vi "CCD Acquire Spectrum vs Wavelength.vi"(11 "error in":errorcluster) -> (15 "error out":errorcluster)   [LabVIEW 2020, in "Examples.lvlib"]
doc: "Example for a CCD spectrum acquisition."
uses:
  Examples.lvlib
  4aef6941-9f58-45d1-a797-2b486d7897ac.vi
  Classes/CCD/CCD.lvclass
  Classes/Mono/Monochromator.lvclass
  <userlib>/_OpenG.lib/error/error.llb/openg_error.lvlib
  <vilib>/Utility/file.llb/Write Delimited Spreadsheet (DBL).vi
panel:
  out "new wavelength":dbl format="%.2f"
  out "XY Graph":cluster{"xAxis":dbl[], "imageData":dbl[]}(graph)
  # "Connector Pane"
  # "Locals"
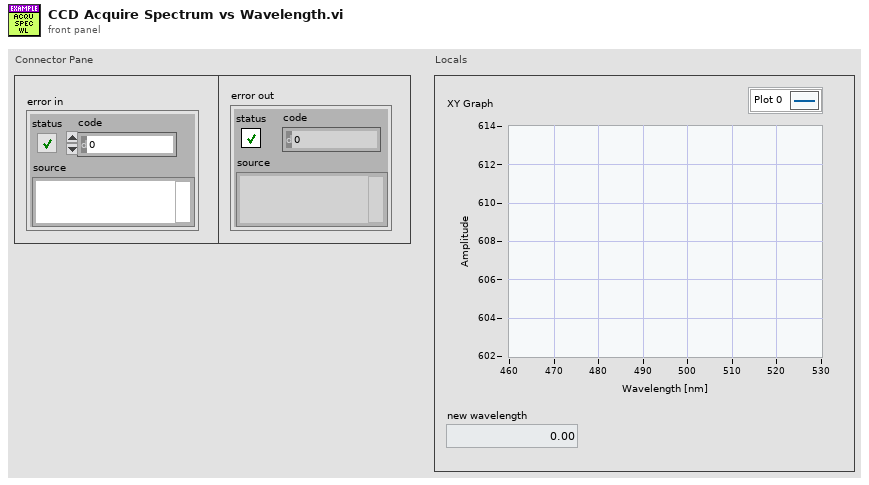
[diagram p1: front panel]
types:
  T1 = cluster{"ROI-index":i32, "xOrigin":i32, "yOrigin":i32, "xSize":i32, "ySize":i32, "xBin":i32, "yBin":i32}
  T2 = typedef "horiba.lvlib/CCD.lvclass/ccdAcquisitionData.ctl" = cluster{"acqIndex":i32, "ROIs":T3[], "timestamp":string}
  T3 = typedef "horiba.lvlib/CCD.lvclass/imageAcqData.ctl" = cluster{"roiMetaData":T4, "xAxis":dbl[], "yData":dbl[][]}
  T4 = typedef "horiba.lvlib/CCD.lvclass/roiMetaData.ctl" = cluster{"roiIndex":i32, "xBinning":i32, "xOrigin":i32, "xSize":i32, "yBinning":i32, "yOrigin":i32, "ySize":i32}
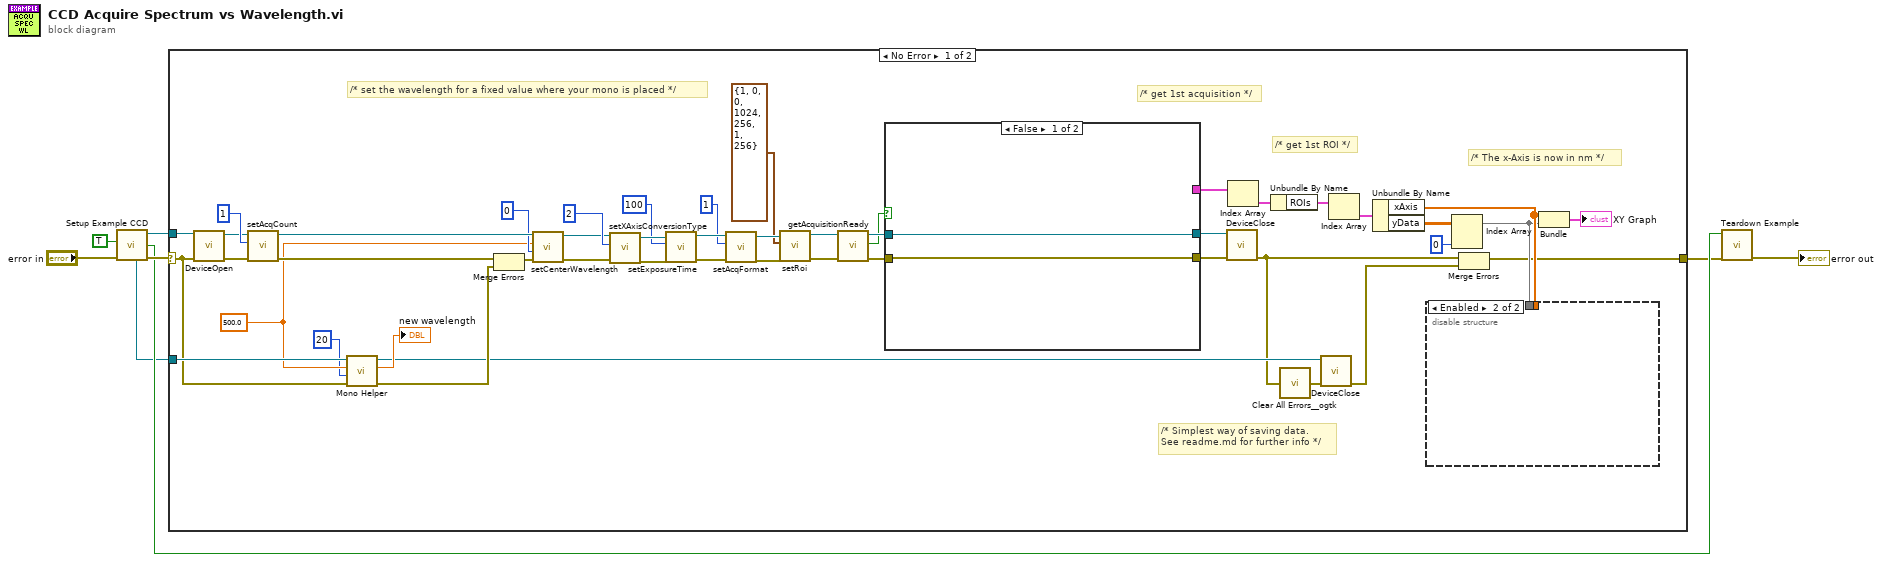
[diagram p0: block diagram]
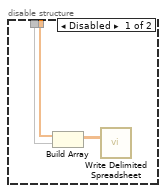
[diagram p2: hidden frame]
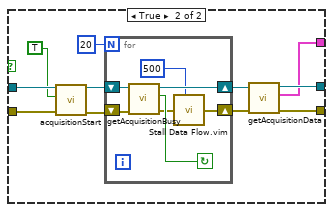
[diagram p3: hidden frame]
diagram:
  n1 = call "Setup Example CCD.vi"("error in (no error)"="error in", "show ICL for debugging"=TRUE) -> ("error out"=w6:errorcluster, "Module Was Already Running?"=w4:bool, "CCD out"=w5:refnum<class "CCD.lvclass">, "Mono out"=w1:refnum<class "Monochromator.lvclass">)  [unwired: 6 in]
  n2 = case shown="No Error" w6 {
    selector: w6 -> [w20 w79]
    tunnel: w5 -> [w32 _]
    tunnel: [w13 w79] -> w3
    tunnel: w1 -> [w21 _]
    frame No Error {
      w10 = 500.0 ("wavelength")
      # "/* set the wavelength for a fixed value where your mono is placed */"
      # "/* The x-Axis is now in nm */"
      # "/* Simplest way of saving data.\nSee readme.md for further info */"
      # "/* get 1st ROI */"
      # "/* get 1st acquisition */"
      n3 = call-dynamic "DeviceOpen.vi"("error in (no error)"=w20, "CCD in"=w32) -> ("error out"=w33:errorcluster, "CCD out"=w31:refnum<class "CCD.lvclass">)  [unwired: 6 in, 2 out]
      n4 = call "setAcqCount.vi"("error in (no error)"=w33, "count"=1, "CCD in"=w31) -> ("error out"=w18:errorcluster, "CCD out"=w26:refnum<class "CCD.lvclass">)  [unwired: 5 in, 2 out]
      n5 = call "Mono Helper.vi"("error in (no error)"=w20, "no of iterations before stop"=20, "wavelength in"=w10, "Monochromator in"=w21) -> ("error out"=w16:errorcluster, "wavelength out"=→"new wavelength":dbl, "Monochromator out"=w15:refnum<class "Monochromator.lvclass">)  [unwired: 5 in]
      n6 = Merge Errors(w18, w16) -> (w17:errorcluster)
      n7 = call "setCenterWavelength.vi"("error in (no error)"=w17, "monoIndex"=0, "wavelength"=w10, "CCD in"=w26) -> ("error out"=w27:errorcluster, "CCD out"=w25:refnum<class "CCD.lvclass">)  [unwired: 4 in, 2 out]
      n8 = call "setXAxisConversionType.vi"("error in (no error)"=w27, "type"=2, "CCD in"=w25) -> ("error out"=w53:errorcluster, "CCD out"=w52:refnum<class "CCD.lvclass">)  [unwired: 5 in, 2 out]
      n9 = call "setExposureTime.vi"("error in (no error)"=w53, "exposure time [ms] or [us]"=100, "CCD in"=w52) -> ("error out"=w50:errorcluster, "CCD out"=w49:refnum<class "CCD.lvclass">)  [unwired: 5 in, 2 out]
      n10 = call "setAcqFormat.vi"("error in (no error)"=w50, "number of ROIs"=1, "CCD in"=w49) -> ("error out"=w47:errorcluster, "CCD out"=w46:refnum<class "CCD.lvclass">)  [unwired: 5 in, 2 out]
      n11 = call "setRoi.vi"("error in (no error)"=w47, "roiConfig"=T1 {"ROI-index"=1, "xOrigin"=0, "yOrigin"=0, "xSize"=1024, "ySize"=256, "xBin"=1, "yBin"=256}, "CCD in"=w46) -> ("error out"=w45:errorcluster, "CCD out"=w28:refnum<class "CCD.lvclass">)  [unwired: 5 in, 2 out]
      n12 = call "getAcquisitionReady.vi"("error in (no error)"=w45, "CCD in"=w28) -> ("error out"=w44:errorcluster, "ready"=w42:bool, "CCD out"=w43:refnum<class "CCD.lvclass">)  [unwired: 7 in]
      n13 = case shown="False" w42 {
        tunnel: w44 -> [w59 w71]
        tunnel: w43 -> [w60 w70]
        tunnel: [w59 w64] -> w41
        tunnel: [w60 w62] -> w40
        tunnel: [_ w61] -> w38
        frame False {
        }
        frame True {
          n14 = call "acquisitionStart.vi"("error in (no error)"=w71, "openShutter"=TRUE, "CCD in"=w70) -> ("error out"=w66:errorcluster, "CCD out"=w65:refnum<class "CCD.lvclass">)  [unwired: 5 in, 2 out]
          n15 = for {
            N: 20 -> [_]
            shift-right: [w74] -> w67
            shift-left: w66 -> [w77]
            shift-right: [w73] -> w63
            shift-left: w65 -> [w78]
            stop <- w76 continue-if-true
            n16 = call "getAcquisitionBusy.vi"("error in (no error)"=w77, "CCD in"=w78) -> ("error out"=w75:errorcluster, "isBusy"=w76:bool, "CCD out"=w73:refnum<class "CCD.lvclass">)  [unwired: 7 in]
            n17 = call "Stall Data Flow.vim"("value in"=w75, "milliseconds to wait"=u32 500) -> ("value out"=w74:errorcluster)  [unwired: 1 out]
          }
          n18 = call "getAcquisitionData.vi"("error in (no error)"=w67, "CCD in"=w63) -> ("error out"=w64:errorcluster, "ccdAcquisitions"=w61:T2[], "CCD out"=w62:refnum<class "CCD.lvclass">)  [unwired: 6 in, 1 out]
        }
      }
      n19 = call-dynamic "DeviceClose.vi"("error in (no error)"=w41, "CCD in"=w40) -> ("error out"=w14:errorcluster)  [unwired: 5 in, 4 out]
      n20 = Index Array(array=w38) -> (element=w37:T2)  [unwired: 1 in]
      n21 = Unbundle By Name(w37) -> ("ROIs"=w36:T3[])
      n22 = call <userlib>:"Clear All Errors__ogtk.vi"("Error In"=w14) -> ("Error Out"=w11:errorcluster)  [unwired: 3 in]
      n23 = call-dynamic "DeviceClose.vi"("error in (no error)"=w11, "Monochromator in"=w15) -> ("error out"=w12:errorcluster)  [unwired: 5 in, 4 out]
      n24 = Index Array(array=w36) -> (element=w35:T3)  [unwired: 1 in]
      n25 = Unbundle By Name(w35) -> ("xAxis"=w30:dbl[], "yData"=w29:dbl[][])
      n26 = Index Array(array=w29, index (col)=0 ("disabled index (col)")) -> (element=w23:dbl[])  [unwired: 1 in]
      n27 = disable-structure shown="Enabled" {
        disable-tunnel: w30 -> [w58 _]
        disable-tunnel: w23 -> [w57 _]
        frame Disabled {
          n28 = Build Array(w58, w57) -> (w56:dbl[][])
          n29 = call-poly <vilib>:"Write Delimited Spreadsheet.vi"("2D data"=w56) -> ()  [unwired: 13 in, 2 out]
        }
        frame Enabled {
        }
      }
      n30 = Merge Errors(w14, w12) -> (w13:errorcluster)
      n31 = Bundle("xAxis"=w30, "yData"=w23) -> (→"XY Graph":cluster{"xAxis":dbl[], "yData":dbl[]})  [unwired: 1 in]
    }
    frame Error {
    }
  }
  n32 = call "Teardown Example.vi"("error in (no error)"=w3, "Module Was Already Running?"=w4) -> ("error out"=→"error out":errorcluster)  [unwired: 9 in]
